vi "modbus_Puck.vi"(6 "Параметры":T3, 8 "Error In":errorcluster, 9 "Pair in":T1={"Давление заданное"=0.3, "Давление в системе"=99.99, "Расход заданый"=0.0, "Расход текущий"=0.0, "Объём заданный"=0.0, "Объём текущий"=0.0, "Старт давление"=FALSE, "Старт расход"=FALSE, "Сброс объёма"=FALSE, "plc_control"=FALSE, "lag_control"=FALSE, "mstop_control"=FALSE, "Давление"={"АЦП CH 0"=0.0, "АЦП CH 1"=0.0, "АЦП CH 2"=0.0, "АЦП CH 3"=0.0, "АЦП CH 4"=0.0, "АЦП CH 5"=0.0, "АЦП CH 6"=0.0, "АЦП CH 7"=0.0}, "Modbus"={"Массив чтения"=[], "Массив записи"=[]}} {"Давление"."АЦП CH 7" format="%.3f"; "Давление"."АЦП CH 6" format="%.3f"; "Давление"."АЦП CH 5" format="%.3f"; "Давление"."АЦП CH 4" format="%.3f"; "Давление"."АЦП CH 3" format="%.3f"; "Давление"."АЦП CH 2" format="%.3f"; "Давление"."АЦП CH 1" format="%.3f"; "Давление"."АЦП CH 0" format="%.3f"; "Объём текущий" min=0.0 max=9999.0 step=0.0001 format="%#_5f"; "Объём заданный" min=0.0 max=9999.0 step=0.0001 format="%#_5f"; "Расход текущий" format="%#_5f"; "Расход заданый" min=0.0 max=40.0 step=0.0001 format="%#_5f"; "Давление в системе" format="%.3f"; "Давление заданное" min=0.3 max=100.0 step=0.01 format="%#_5f"}, 10 "Port 2 in":T2={"Давление заданное"=0.3, "Давление MAX заданное"=100.0, "Давление в насосе"=0.0, "Давление в системе"=99.99, "Расход заданый"=0.0, "Расход текущий"=0.0, "Объём заданный"=0.0, "Объём текущий"=0.0, "Позиция насоса %"=0.0, "Ток двигателя"=0.0, "controlMsg"="", "Клапан k_sys"=FALSE, "Клапан k_res"=FALSE, "Клапан k_air"=FALSE, "Вверх"=FALSE, "Домой"=FALSE, "Вниз"=FALSE, "Старт расход"=FALSE, "Старт давление"=FALSE, "Сброс объёма"=FALSE, "Сброс давления Рсис"=FALSE, "Сброс давления Рнас"=FALSE, "Bits"={"plc_control"=FALSE, "lag_control"=FALSE, "mstop_control"=FALSE, "st_home"=FALSE, "error"=FALSE, "mstart"=FALSE, "pair"=FALSE, "startQ"=FALSE, "startP"=FALSE, "volume_Stop"=FALSE}} {"Ток двигателя" format="%#_5f"; "Расход текущий" format="%#_5f"; "Давление в системе" format="%.3f"; "Объём текущий" min=0.0 max=9999.0 step=0.0001 format="%#_5f"; "Объём заданный" min=0.0 max=9999.0 step=0.0001 format="%#_5f"; "Давление MAX заданное" min=0.0 max=100.0 step=0.01 format="%#_5f"; "Давление заданное" min=0.3 max=100.0 step=0.01 format="%#_5f"; "Расход заданый" min=0.0 max=40.0 step=0.0001 format="%#_5f"; "Давление в насосе" format="%.3f"; "Позиция насоса %" scale=0.0..100.0 scale format="%.2f"}, 11 "Port 1 in":T2={"Давление заданное"=0.3, "Давление MAX заданное"=100.0, "Давление в насосе"=0.0, "Давление в системе"=99.99, "Расход заданый"=0.0, "Расход текущий"=0.0, "Объём заданный"=0.0, "Объём текущий"=0.0, "Позиция насоса %"=0.0, "Ток двигателя"=0.0, "controlMsg"="", "Клапан k_sys"=FALSE, "Клапан k_res"=FALSE, "Клапан k_air"=FALSE, "Вверх"=FALSE, "Домой"=FALSE, "Вниз"=FALSE, "Старт расход"=FALSE, "Старт давление"=FALSE, "Сброс объёма"=FALSE, "Сброс давления Рсис"=FALSE, "Сброс давления Рнас"=FALSE, "Bits"={"plc_control"=FALSE, "lag_control"=FALSE, "mstop_control"=FALSE, "st_home"=FALSE, "error"=FALSE, "mstart"=FALSE, "pair"=FALSE, "startQ"=FALSE, "startP"=FALSE, "volume_Stop"=FALSE}} {"Ток двигателя" format="%#_5f"; "Расход текущий" format="%#_5f"; "Давление в системе" format="%.3f"; "Объём текущий" min=0.0 max=9999.0 step=0.0001 format="%#_5f"; "Объём заданный" min=0.0 max=9999.0 step=0.0001 format="%#_5f"; "Давление MAX заданное" min=0.0 max=100.0 step=0.01 format="%#_5f"; "Давление заданное" min=0.3 max=100.0 step=0.01 format="%#_5f"; "Расход заданый" min=0.0 max=40.0 step=0.0001 format="%#_5f"; "Давление в насосе" format="%.3f"; "Позиция насоса %" scale=0.0..100.0 scale format="%.2f"}) -> (0 "Error Out":errorcluster, 1 "Pair out":T1={"Давление заданное"=0.3, "Давление в системе"=99.99, "Расход заданый"=0.0, "Расход текущий"=0.0, "Объём заданный"=0.0, "Объём текущий"=0.0, "Старт давление"=FALSE, "Старт расход"=FALSE, "Сброс объёма"=FALSE, "plc_control"=FALSE, "lag_control"=FALSE, "mstop_control"=FALSE, "Давление"={"АЦП CH 0"=0.0, "АЦП CH 1"=0.0, "АЦП CH 2"=0.0, "АЦП CH 3"=0.0, "АЦП CH 4"=0.0, "АЦП CH 5"=0.0, "АЦП CH 6"=0.0, "АЦП CH 7"=0.0}, "Modbus"={"Массив чтения"=[], "Массив записи"=[]}} {"Давление"."АЦП CH 7" format="%.3f"; "Давление"."АЦП CH 6" format="%.3f"; "Давление"."АЦП CH 5" format="%.3f"; "Давление"."АЦП CH 4" format="%.3f"; "Давление"."АЦП CH 3" format="%.3f"; "Давление"."АЦП CH 2" format="%.3f"; "Давление"."АЦП CH 1" format="%.3f"; "Давление"."АЦП CH 0" format="%.3f"; "Объём текущий" min=0.0 max=9999.0 step=0.0001 format="%#_5f"; "Объём заданный" min=0.0 max=9999.0 step=0.0001 format="%#_5f"; "Расход текущий" format="%#_5f"; "Расход заданый" min=0.0 max=40.0 step=0.0001 format="%#_5f"; "Давление в системе" format="%.3f"; "Давление заданное" min=0.3 max=100.0 step=0.01 format="%#_5f"}, 2 "Port 2 out":T2={"Давление заданное"=0.3, "Давление MAX заданное"=100.0, "Давление в насосе"=0.0, "Давление в системе"=99.99, "Расход заданый"=0.0, "Расход текущий"=0.0, "Объём заданный"=0.0, "Объём текущий"=0.0, "Позиция насоса %"=0.0, "Ток двигателя"=0.0, "controlMsg"="", "Клапан k_sys"=FALSE, "Клапан k_res"=FALSE, "Клапан k_air"=FALSE, "Вверх"=FALSE, "Домой"=FALSE, "Вниз"=FALSE, "Старт расход"=FALSE, "Старт давление"=FALSE, "Сброс объёма"=FALSE, "Сброс давления Рсис"=FALSE, "Сброс давления Рнас"=FALSE, "Bits"={"plc_control"=FALSE, "lag_control"=FALSE, "mstop_control"=FALSE, "st_home"=FALSE, "error"=FALSE, "mstart"=FALSE, "pair"=FALSE, "startQ"=FALSE, "startP"=FALSE, "volume_Stop"=FALSE}} {"Ток двигателя" format="%#_5f"; "Расход текущий" format="%#_5f"; "Давление в системе" format="%.3f"; "Объём текущий" min=0.0 max=9999.0 step=0.0001 format="%#_5f"; "Объём заданный" min=0.0 max=9999.0 step=0.0001 format="%#_5f"; "Давление MAX заданное" min=0.0 max=100.0 step=0.01 format="%#_5f"; "Давление заданное" min=0.3 max=100.0 step=0.01 format="%#_5f"; "Расход заданый" min=0.0 max=40.0 step=0.0001 format="%#_5f"; "Давление в насосе" format="%.3f"; "Позиция насоса %" scale=0.0..100.0 scale format="%.2f"}, 3 "Port 1 out":T2={"Давление заданное"=0.3, "Давление MAX заданное"=100.0, "Давление в насосе"=0.0, "Давление в системе"=99.99, "Расход заданый"=0.0, "Расход текущий"=0.0, "Объём заданный"=0.0, "Объём текущий"=0.0, "Позиция насоса %"=0.0, "Ток двигателя"=0.0, "controlMsg"="", "Клапан k_sys"=FALSE, "Клапан k_res"=FALSE, "Клапан k_air"=FALSE, "Вверх"=FALSE, "Домой"=FALSE, "Вниз"=FALSE, "Старт расход"=FALSE, "Старт давление"=FALSE, "Сброс объёма"=FALSE, "Сброс давления Рсис"=FALSE, "Сброс давления Рнас"=FALSE, "Bits"={"plc_control"=FALSE, "lag_control"=FALSE, "mstop_control"=FALSE, "st_home"=FALSE, "error"=FALSE, "mstart"=FALSE, "pair"=FALSE, "startQ"=FALSE, "startP"=FALSE, "volume_Stop"=FALSE}} {"Ток двигателя" format="%#_5f"; "Расход текущий" format="%#_5f"; "Давление в системе" format="%.3f"; "Объём текущий" min=0.0 max=9999.0 step=0.0001 format="%#_5f"; "Объём заданный" min=0.0 max=9999.0 step=0.0001 format="%#_5f"; "Давление MAX заданное" min=0.0 max=100.0 step=0.01 format="%#_5f"; "Давление заданное" min=0.3 max=100.0 step=0.01 format="%#_5f"; "Расход заданый" min=0.0 max=40.0 step=0.0001 format="%#_5f"; "Давление в насосе" format="%.3f"; "Позиция насоса %" scale=0.0..100.0 scale format="%.2f"}, 5 "Modbus Write":u16[](array[numeric]))   [LabVIEW 2023, in "pump_Lib.lvlib"]
uses:
  pump_Lib.lvlib
  TypeDef/pump_Type.ctl
  TypeDef/parametrs_Type.ctl
  TypeDef/pair_Type.ctl
  <vilib>/ptbypt/NI_PtbyPt.lvlib
panel:
  out "last write":dbl format="%_19f"
  # "%"
  # "%"
  # "%"
  # "%"
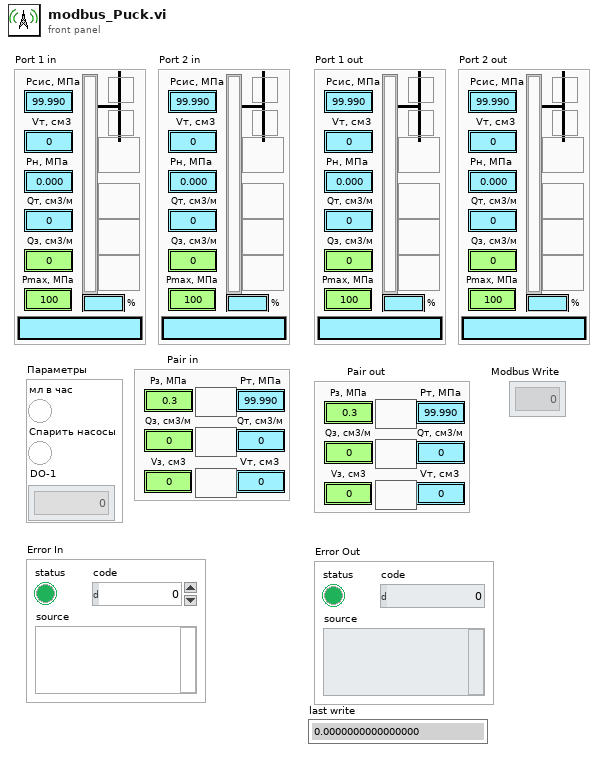
[diagram p1: front panel]
types:
  T1 = typedef "pump_Lib.lvlib/pair_Type.ctl" = cluster{"Давление заданное":dbl, "Давление в системе":dbl, "Расход заданый":dbl, "Расход текущий":dbl, "Объём заданный":dbl, "Объём текущий":dbl, "Старт давление":bool, "Старт расход":bool, "Сброс объёма":bool, "plc_control":bool, "lag_control":bool, "mstop_control":bool, "Давление":cluster{"АЦП CH 0":dbl, "АЦП CH 1":dbl, "АЦП CH 2":dbl, "АЦП CH 3":dbl, "АЦП CH 4":dbl, "АЦП CH 5":dbl, "АЦП CH 6":dbl, "АЦП CH 7":dbl}, "Modbus":cluster{"Массив чтения":u16[], "Массив записи":u16[]}}
  T2 = typedef "pump_Lib.lvlib/pump_Type.ctl" = cluster{"Давление заданное":dbl, "Давление MAX заданное":dbl, "Давление в насосе":dbl, "Давление в системе":dbl, "Расход заданый":dbl, "Расход текущий":dbl, "Объём заданный":dbl, "Объём текущий":dbl, "Позиция насоса %":dbl, "Ток двигателя":dbl, "controlMsg":string, "Клапан k_sys":bool, "Клапан k_res":bool, "Клапан k_air":bool, "Вверх":bool, "Домой":bool, "Вниз":bool, "Старт расход":bool, "Старт давление":bool, "Сброс объёма":bool, "Сброс давления Рсис":bool, "Сброс давления Рнас":bool, "Bits":cluster{"plc_control":bool, "lag_control":bool, "mstop_control":bool, "st_home":bool, "error":bool, "mstart":bool, "pair":bool, "startQ":bool, "startP":bool, "volume_Stop":bool}}
  T3 = typedef "pump_Lib.lvlib/parametrs_Type.ctl" = cluster{"мл в час":bool, "Спарить насосы":bool, "DO-1":u16[]}
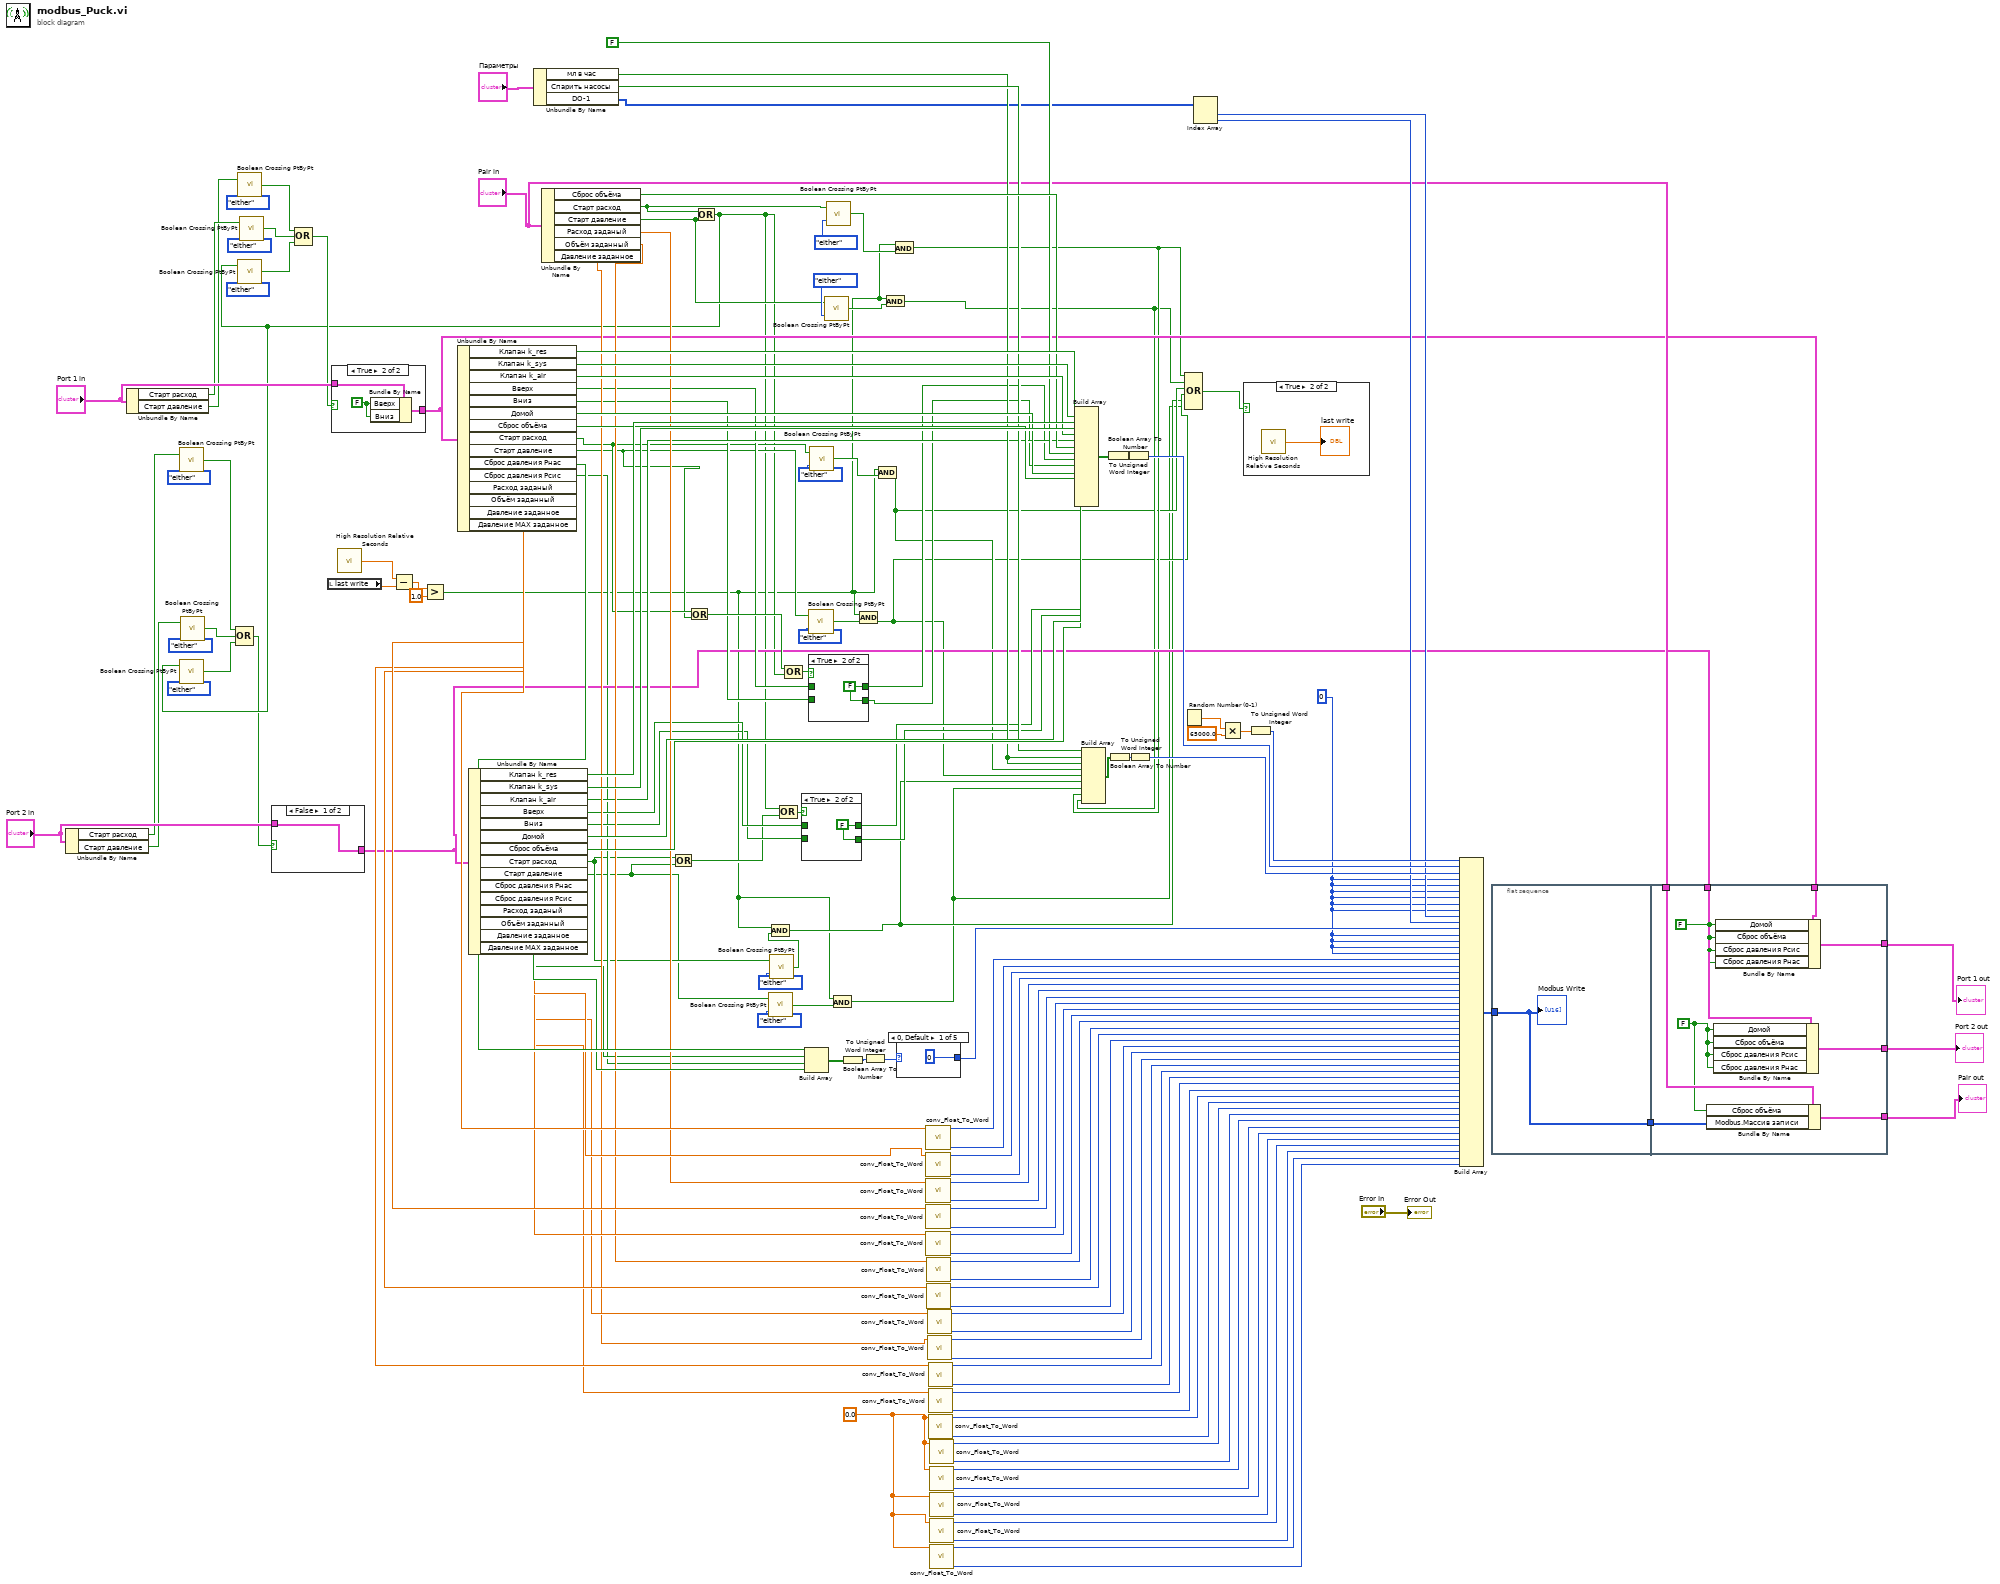
[diagram p0: block diagram]
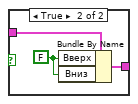
[diagram p3: hidden frame]
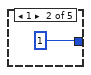
[diagram p7: hidden frame]
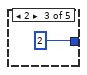
[diagram p8: hidden frame]
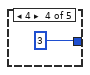
[diagram p9: hidden frame]
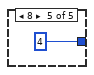
[diagram p10: hidden frame]
diagram:
  w75 = 0.0
  w43 = u16 0 ("value")
  n1 = Unbundle By Name("Port 2 in") -> ("Старт расход"=w20:bool, "Старт давление"=w19:bool)
  n2 = Unbundle By Name("Port 1 in") -> ("Старт расход"=w33:bool, "Старт давление"=w32:bool)
  n3 = call <vilib>:"Boolean Crossing PtByPt.vi"("direction"=enum16{"either", "false-true", "true-false"}."either", "input"=w20) -> ("crossing"=w25:bool)  [unwired: 1 in]
  n4 = call <vilib>:"Boolean Crossing PtByPt.vi"("direction"=enum16{"either", "false-true", "true-false"}."either", "input"=w19) -> ("crossing"=w26:bool)  [unwired: 1 in]
  n5 = call <vilib>:"Boolean Crossing PtByPt.vi"("direction"=enum16{"either", "false-true", "true-false"}."either", "input"=w32) -> ("crossing"=w31:bool)  [unwired: 1 in]
  n6 = call <vilib>:"Boolean Crossing PtByPt.vi"("direction"=enum16{"either", "false-true", "true-false"}."either", "input"=w33) -> ("crossing"=w30:bool)  [unwired: 1 in]
  n7 = local read "last write"() -> (w4:dbl)
  n8 = call <vilib>:"High Resolution Relative Seconds.vi"() -> ("relative seconds"=w5:dbl)
  n9 = Subtract(x=w5, y=w4) -> (x-y=w3:dbl)
  n10 = Greater?(x=w3, y=1.0) -> (0:w1:bool)
  n11 = Unbundle By Name("Параметры") -> ("мл в час"=w130:bool, "Спарить насосы"=w131:bool, "DO-1"=w125:u16[])
  n12 = Unbundle By Name("Pair in") -> ("Сброс объёма"=w137:bool, "Старт расход"=w37:bool, "Старт давление"=w36:bool, "Расход заданый"=w115:dbl, "Объём заданный"=w112:dbl, "Давление заданное"=w109:dbl)
  n13 = Or(x=w37, y=w36) -> (x .or. y?=w21:bool)
  n14 = call <vilib>:"Boolean Crossing PtByPt.vi"("direction"=enum16{"either", "false-true", "true-false"}."either", "input"=w21) -> ("crossing"=w27:bool)  [unwired: 1 in]
  n15 = Compound Arithmetic op=OR(w25, w26, w27) -> (w18:bool)
  n16 = call <vilib>:"Boolean Crossing PtByPt.vi"("direction"=enum16{"either", "false-true", "true-false"}."either", "input"=w21) -> ("crossing"=w29:bool)  [unwired: 1 in]
  n17 = case shown="False" w18 {
    tunnel: "Port 2 in" -> [w156 w159]
    tunnel: [w156 w157] -> w51
    frame False {
    }
    frame True {
      w158 = FALSE ("Вверх")
      n18 = Bundle By Name(cluster=w159, "Вверх"=w158, "Вниз"=w158) -> (w157:T2)
    }
  }
  n19 = Compound Arithmetic op=OR(w31, w30, w29) -> (w28:bool)
  n20 = case shown="True" w28 {
    tunnel: "Port 1 in" -> [w160 w163]
    tunnel: [w160 w161] -> w53
    frame False {
    }
    frame True {
      w162 = FALSE ("Вверх")
      n21 = Bundle By Name(cluster=w163, "Вверх"=w162, "Вниз"=w162) -> (w161:T2)
    }
  }
  n22 = Unbundle By Name(w53) -> ("Клапан k_res"=w142:bool, "Клапан k_sys"=w141:bool, "Клапан k_air"=w138:bool, "Вверх"=w59:bool, "Вниз"=w57:bool, "Домой"=w135:bool, "Сброс объёма"=w134:bool, "Старт расход"=w47:bool, "Старт давление"=w46:bool, "Сброс давления Рнас"=w122:bool, "Сброс давления Рсис"=w49:bool, "Расход заданый"=w117:dbl, "Объём заданный"=w114:dbl, "Давление заданное"=w111:dbl, "Давление MAX заданное"=w108:dbl)
  n23 = Unbundle By Name(w51) -> ("Клапан k_res"=w140:bool, "Клапан k_sys"=w139:bool, "Клапан k_air"=w62:bool, "Вверх"=w68:bool, "Вниз"=w66:bool, "Домой"=w133:bool, "Сброс объёма"=w132:bool, "Старт расход"=w39:bool, "Старт давление"=w38:bool, "Сброс давления Рнас"=w50:bool, "Сброс давления Рсис"=w121:bool, "Расход заданый"=w116:dbl, "Объём заданный"=w113:dbl, "Давление заданное"=w110:dbl, "Давление MAX заданное"=w107:dbl)
  n24 = Or(x=w39, y=w38) -> (x .or. y?=w61:bool)
  n25 = Or(x=w47, y=w46) -> (x .or. y?=w60:bool)
  n26 = call <vilib>:"Boolean Crossing PtByPt.vi"("direction"=enum16{"either", "false-true", "true-false"}."either", "input"=w38) -> ("crossing"=w40:bool)  [unwired: 1 in]
  n27 = call <vilib>:"Boolean Crossing PtByPt.vi"("direction"=enum16{"either", "false-true", "true-false"}."either", "input"=w39) -> ("crossing"=w17:bool)  [unwired: 1 in]
  n28 = And(x=w1, y=w17) -> (x .and. y?=w7:bool)
  n29 = Compound Arithmetic op=OR(w21, w61) -> (w64:bool)
  n30 = Compound Arithmetic op=OR(w60, w21) -> (w63:bool)
  n31 = case shown="True" w64 {
    tunnel: w68 -> [w165 _]
    tunnel: [w165 w166] -> w67
    tunnel: w66 -> [w164 _]
    tunnel: [w164 w166] -> w65
    frame False {
    }
    frame True {
      w166 = FALSE ("Вверх")
    }
  }
  n32 = Build Array(w122, w50, w49, w121) -> (w129:bool[])
  n33 = case shown="True" w63 {
    tunnel: w59 -> [w168 _]
    tunnel: [w168 w169] -> w58
    tunnel: w57 -> [w167 _]
    tunnel: [w167 w169] -> w56
    frame False {
    }
    frame True {
      w169 = FALSE ("Вверх")
    }
  }
  n34 = call <vilib>:"Boolean Crossing PtByPt.vi"("direction"=enum16{"either", "false-true", "true-false"}."either", "input"=w46) -> ("crossing"=w15:bool)  [unwired: 1 in]
  n35 = call <vilib>:"Boolean Crossing PtByPt.vi"("direction"=enum16{"either", "false-true", "true-false"}."either", "input"=w47) -> ("crossing"=w16:bool)  [unwired: 1 in]
  n36 = call <vilib>:"Boolean Crossing PtByPt.vi"("direction"=enum16{"either", "false-true", "true-false"}."either", "input"=w36) -> ("crossing"=w13:bool)  [unwired: 1 in]
  n37 = call <vilib>:"Boolean Crossing PtByPt.vi"("direction"=enum16{"either", "false-true", "true-false"}."either", "input"=w37) -> ("crossing"=w14:bool)  [unwired: 1 in]
  n38 = And(x=w1, y=w40) -> (x .and. y?=w6:bool)
  n39 = Boolean Array To Number(Boolean array=w129) -> (number=w128:u32)
  n40 = And(x=w1, y=w15) -> (x .and. y?=w8:bool)
  n41 = To Unsigned Word Integer(number=w128) -> (unsigned 16bit integer=w127:u16)
  n42 = And(x=w1, y=w16) -> (x .and. y?=w9:bool)
  n43 = And(x=w1, y=w13) -> (x .and. y?=w10:bool)
  n44 = And(x=w1, y=w14) -> (x .and. y?=w12:bool)
  n45 = case shown="0, Default" w127 {
    tunnel: [u16 0 ("lo(x)") u16 1 ("lo(x)") u16 2 ("lo(x)") u16 3 ("lo(x)") u16 4 ("lo(x)")] -> w120
    frame 0, Default {
    }
    frame 1 {
    }
    frame 2 {
    }
    frame 4 {
    }
    frame 8 {
    }
  }
  n46 = call "conv_Float_To_Word.vi"("input_Float"=w117) -> ("second_Word"=w144:u16, "first_Word"=w145:u16)  [unwired: 9 in]
  n47 = call "conv_Float_To_Word.vi"("input_Float"=w116) -> ("second_Word"=w118:u16, "first_Word"=w119:u16)  [unwired: 9 in]
  n48 = call "conv_Float_To_Word.vi"("input_Float"=w115) -> ("second_Word"=w104:u16, "first_Word"=w105:u16)  [unwired: 9 in]
  n49 = call "conv_Float_To_Word.vi"("input_Float"=w114) -> ("second_Word"=w102:u16, "first_Word"=w103:u16)  [unwired: 9 in]
  n50 = call "conv_Float_To_Word.vi"("input_Float"=w113) -> ("second_Word"=w100:u16, "first_Word"=w101:u16)  [unwired: 9 in]
  n51 = call "conv_Float_To_Word.vi"("input_Float"=w112) -> ("second_Word"=w98:u16, "first_Word"=w99:u16)  [unwired: 9 in]
  n52 = call "conv_Float_To_Word.vi"("input_Float"=w111) -> ("second_Word"=w96:u16, "first_Word"=w97:u16)  [unwired: 9 in]
  n53 = call "conv_Float_To_Word.vi"("input_Float"=w110) -> ("second_Word"=w94:u16, "first_Word"=w95:u16)  [unwired: 9 in]
  n54 = call "conv_Float_To_Word.vi"("input_Float"=w109) -> ("second_Word"=w92:u16, "first_Word"=w93:u16)  [unwired: 9 in]
  n55 = call "conv_Float_To_Word.vi"("input_Float"=w108) -> ("second_Word"=w90:u16, "first_Word"=w91:u16)  [unwired: 9 in]
  n56 = call "conv_Float_To_Word.vi"("input_Float"=w107) -> ("second_Word"=w88:u16, "first_Word"=w89:u16)  [unwired: 9 in]
  n57 = call "conv_Float_To_Word.vi"("input_Float"=w75) -> ("second_Word"=w86:u16, "first_Word"=w87:u16)  [unwired: 9 in]
  n58 = call "conv_Float_To_Word.vi"("input_Float"=w75) -> ("second_Word"=w84:u16, "first_Word"=w85:u16)  [unwired: 9 in]
  n59 = call "conv_Float_To_Word.vi"("input_Float"=w75) -> ("second_Word"=w82:u16, "first_Word"=w83:u16)  [unwired: 9 in]
  n60 = call "conv_Float_To_Word.vi"("input_Float"=w75) -> ("second_Word"=w80:u16, "first_Word"=w81:u16)  [unwired: 9 in]
  n61 = call "conv_Float_To_Word.vi"("input_Float"=w75) -> ("second_Word"=w78:u16, "first_Word"=w79:u16)  [unwired: 9 in]
  n62 = call "conv_Float_To_Word.vi"("input_Float"=w75) -> ("second_Word"=w76:u16, "first_Word"=w77:u16)  [unwired: 9 in]
  n63 = Build Array(w142, w141, w140, w139, w138, w62, w137, FALSE, w58, w56, w135, w134, w67, w65, w133, w132) -> (w151:bool[])
  n64 = Build Array(w131, w130, w130, w9, w8, w7, w6, w12, w10) -> (w148:bool[])
  n65 = Boolean Array To Number(Boolean array=w151) -> (number=w150:u32)
  n66 = Boolean Array To Number(Boolean array=w148) -> (number=w149:u32)
  n67 = To Unsigned Word Integer(number=w150) -> (unsigned 16bit integer=w147:u16)
  n68 = To Unsigned Word Integer(number=w149) -> (unsigned 16bit integer=w146:u16)
  n69 = Random Number (0-1)() -> (number: 0 to 1=w155:dbl)
  n70 = Compound Arithmetic op=OR(w12, w10, w9, w8, w7, w6) -> (w11:bool)
  n71 = Index Array(array=w125) -> (element #1=w124:u16, element #2=w123:u16)  [unwired: 2 in]
  n72 = Multiply(x=w155, y=65000.0) -> (x*y=w153:dbl)
  n73 = case shown="True" w11 {
    frame False {
    }
    frame True {
      n74 = call <vilib>:"High Resolution Relative Seconds.vi"() -> ("relative seconds"=→"last write":dbl)
    }
  }
  n75 = To Unsigned Word Integer(number=w153) -> (unsigned 16bit integer=w152:u16)
  n76 = Build Array(w152, w147, w146, w43, w43, w43, w43, w43, w43, w124, w123, w120, w43, w43, w43, w43, w145, w144, w119, w118, w105, w104, w103, w102, w101, w100, w99, w98, w97, w96, w95, w94, w93, w92, w91, w90, w89, w88, w87, w86, w85, w84, w83, w82, w81, w80, w79, w78, w77, w76) -> (w74:u16[])
  n77 = flat-sequence {
    tunnel: w74 -> [w176]
    tunnel: [w176] -> w72
    tunnel: w53 -> [w185]
    tunnel: w51 -> [w184]
    tunnel: "Pair in" -> [w182]
    tunnel: w72 -> [w180]
    tunnel: [w179] -> w71
    tunnel: [w178] -> w70
    tunnel: [w177] -> w69
    frame #0 {
      "Modbus Write" <- w176
    }
    frame #1 {
      w181 = FALSE ("Домой")
      w183 = FALSE ("Домой")
      n78 = Bundle By Name(cluster=w182, "Сброс объёма"=w181, "Modbus.Массив записи"=w180) -> (w177:T1)
      n79 = Bundle By Name(cluster=w184, "Домой"=w181, "Сброс объёма"=w181, "Сброс давления Рсис"=w181, "Сброс давления Рнас"=w181) -> (w178:T2)
      n80 = Bundle By Name(cluster=w185, "Домой"=w183, "Сброс объёма"=w183, "Сброс давления Рсис"=w183, "Сброс давления Рнас"=w183) -> (w179:T2)
    }
  }
  "Port 1 out" <- w71
  "Port 2 out" <- w70
  "Pair out" <- w69
  "Error Out" <- "Error In"
